vi "Read_XYSens_SR5x10.vi"(9 "Ring":u16(ring) items=["SR 5110", "SR 5210"], 11 "7265 GPIB":string="7") -> (0 "Sen":dbl format="%#_13g", 2 "Yout":dbl format="%#_13g", 3 "Xout":dbl format="%#_13g")   [LabVIEW 2014]
panel:
  out "Xout 2":dbl format="%#_13g"
  out "Yout 2":dbl format="%#_13g"
  out "error out":errorcluster
  in  "error in (no error)":errorcluster
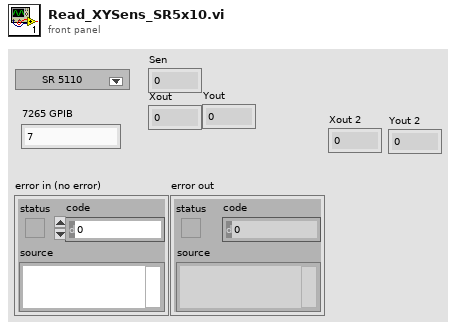
[diagram p1: front panel]
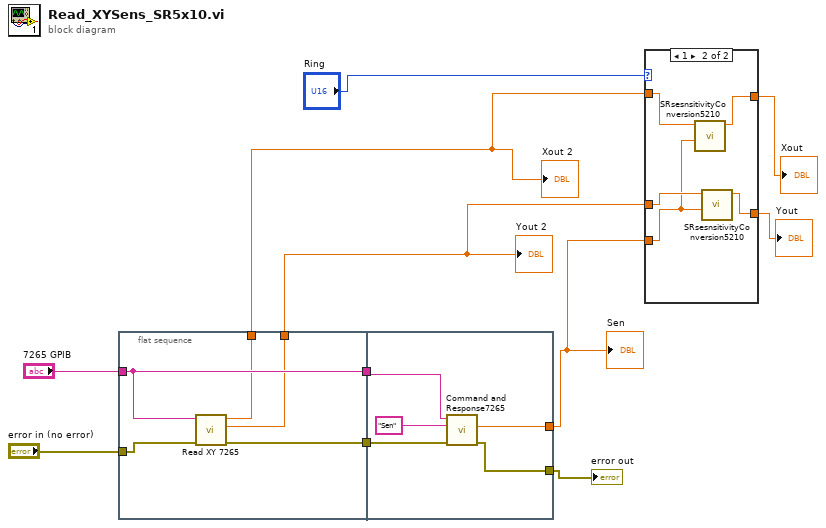
[diagram p0: block diagram]
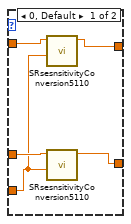
[diagram p2: hidden frame]
diagram:
  n1 = flat-sequence {
    tunnel: "7265 GPIB" -> [w14]
    tunnel: "error in (no error)" -> [w16]
    tunnel: [w15] -> w8
    tunnel: [w14] -> w7
    tunnel: [w13] -> w4
    tunnel: [w12] -> w5
    tunnel: [w20] -> w11
    tunnel: w8 -> [w19]
    tunnel: w7 -> [w18]
    tunnel: [w17] -> w3
    frame #0 {
      n2 = call "Read XY 7265.vi"("error in (no error)"=w16, "7265 GPIB"=w14) -> ("error out"=w15:errorcluster, "Y channel"=w13:dbl, "X channel"=w12:dbl)  [unwired: 7 in]
    }
    frame #1 {
      n3 = call "Command and Response7265.vi"("error in (no error)"=w19, "Command"="Sen", "7265 GPIB"=w18) -> ("error out"=w20:errorcluster, "Response Code Only"=w17:dbl)  [unwired: 6 in, 1 out]
    }
  }
  n4 = case shown="1" "Ring" {
    tunnel: w5 -> [w24 w31]
    tunnel: w4 -> [w26 w30]
    tunnel: w3 -> [w25 w29]
    tunnel: [w23 w28] -> w2
    tunnel: [w22 w27] -> w1
    frame 0, Default {
      n5 = call "SRsesnsitivityConversion5110.vi"("Sen"=w25, "Input"=w24) -> ("Output"=w23:dbl)  [unwired: 9 in]
      n6 = call "SRsesnsitivityConversion5110.vi"("Sen"=w25, "Input"=w26) -> ("Output"=w22:dbl)  [unwired: 9 in]
    }
    frame 1 {
      n7 = call "SRsesnsitivityConversion5210.vi"("Sen"=w29, "Input"=w31) -> ("Output"=w28:dbl)  [unwired: 9 in]
      n8 = call "SRsesnsitivityConversion5210.vi"("Sen"=w29, "Input"=w30) -> ("Output"=w27:dbl)  [unwired: 9 in]
    }
  }
  "Xout" <- w2
  "Yout" <- w1
  "error out" <- w11
  "Sen" <- w3
  "Yout 2" <- w4
  "Xout 2" <- w5
